vi "Init FPGA.vi"(3 "FIFO depth":u32=8000) -> (0 "FPGA error out":errorcluster, 1 "FPGA VI Reference Out":refnum<k20>, 2 "Actual Depth":u32)   [LabVIEW 2014]
uses:
  <vilib>/FPGAPlugInAG/PXI-7854R/niLvFpga_Open_PXI-7854R.vi
  <vilib>/FPGAPlugInAG/PXI-7854R/niLvFpga_Reset_PXI-7854R.vi
  <vilib>/FPGAPlugInAG/PXI-7854R/niLvFpga_Run_PXI-7854R.vi
  <vilib>/Utility/error.llb/Error Cluster From Error Code.vi
  <vilib>/rvi/errors/niLvFpgaAdjustHostInterfaceError.vi
  <vilib>/rvi/interface/common/niFpgaWaitOnOcc.vi
  <vilib>/rvi/interface/nirviOpenFPGA/nirviOpenFPGA.xnode
  FPGA Bitfiles/OmicronR2_FPGATarget_CountertoDAC_vJTICW5rMr0.lvbitx
  FPGA vi/Counter to DAC.vi
  <vilib>/rvi/interface/nirviMethod/nirviMethod.xnode
  <vilib>/rvi/interface/nirviReadWriteControl/nirviReadWriteControl.xnode
  <vilib>/rvi/errors/niLvFpgaMergeErrorWithErrorCode.vi
  NiFpgaLv.dll
  <vilib>/FPGAPlugInAG/PXI-7854R/niLvFpga_ConfigureFifo_PXI-7854R.vi
  <vilib>/FPGAPlugInAG/PXI-7854R/niLvFpga_StartFifo_PXI-7854R.vi
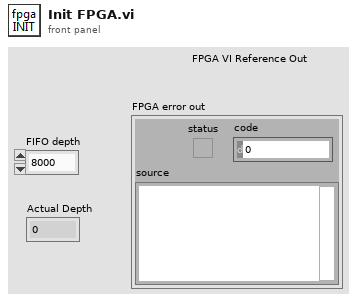
[diagram p1: front panel]
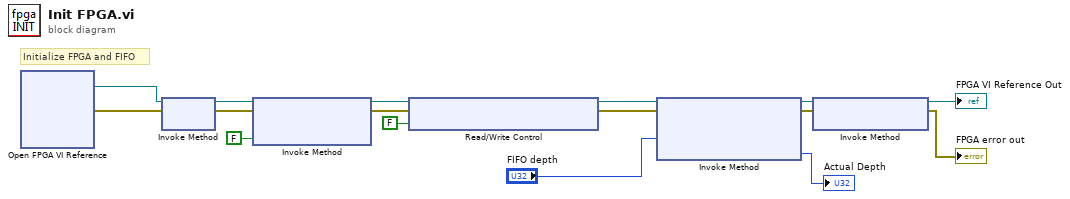
[diagram p0: block diagram]
diagram:
  # "Initialize FPGA and FIFO"
  n1 = xnode "Open FPGA VI Reference"() -> ("FPGA VI Reference Out"=w9:refnum<k20>, "error out"=w10:errorcluster)  [unwired: 2 in]
  n2 = xnode "Invoke Method"("FPGA VI Reference In"=w9, "error in"=w10) -> ("FPGA VI Reference Out"=w11:refnum<k20>, "error out"=w12:errorcluster)
  n3 = xnode "Invoke Method"("FPGA VI Reference In"=w11, "error in"=w12, "Wait Until Done (F)"=FALSE) -> ("FPGA VI Reference Out"=w13:refnum<k20>, "error out"=w14:errorcluster)
  n4 = xnode "Read/Write Control"("FPGA VI Reference In"=w13, "error in"=w14, "Ctr FIFO"=FALSE) -> ("FPGA VI Reference Out"=w4:refnum<k20>, "error out"=w6:errorcluster)
  n5 = xnode "Invoke Method"("FPGA VI Reference In"=w4, "error in"=w6, "Requested Depth"="FIFO depth") -> ("FPGA VI Reference Out"=w5:refnum<k20>, "error out"=w7:errorcluster, "Actual Depth"=→"Actual Depth":u32)
  n6 = xnode "Invoke Method"("FPGA VI Reference In"=w5, "error in"=w7) -> ("FPGA VI Reference Out"=→"FPGA VI Reference Out":refnum<k20>, "error out"=→"FPGA error out":errorcluster)
